vi "ErrorHandler.vi"(6 "EnqueueType (QMH)":T1, 8 "error in (no error)":errorcluster, 11 "Queue Array Reference In":refnum<queue>[](array[refnum])) -> (0 "error out":errorcluster)   [LabVIEW 2018, in "ScopePlugins.lvlib"]
uses:
  ScopePlugins.lvlib
  TypeDefs/QueueNames.ctl
  clMessage.ctl
  EnqueueTypes.ctl
panel:
  in  "Message (Error)":string="Error"
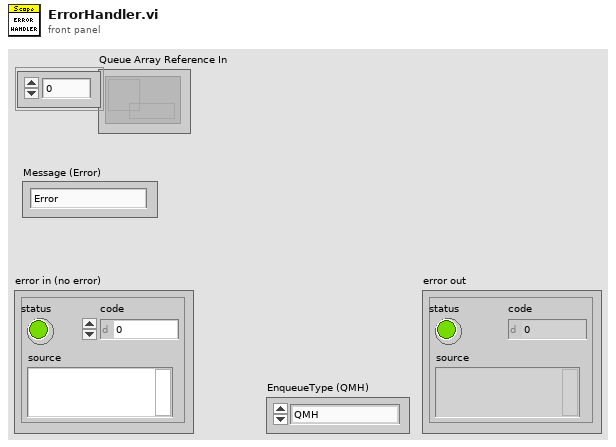
[diagram p1: front panel]
types:
  T1 = typedef "ScopePlugins.lvlib/QueueNames.ctl" = enum16{"QMH", "Class ", "MA"}
  T2 = typedef "ScopePlugins.lvlib/EnqueueTypes.ctl" = enum16{"LossyEnqueue", "EnqueueAtFront", "Enqueue"}
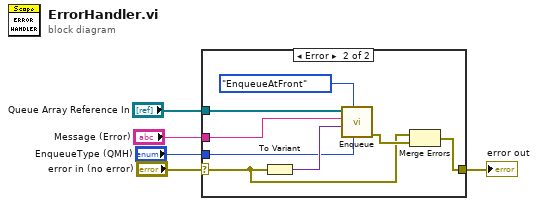
[diagram p0: block diagram]
diagram:
  n1 = case shown="Error" "error in (no error)" {
    selector: "error in (no error)" -> [w6 w7]
    tunnel: "Message (Error)" -> [_ w13]
    tunnel: "Queue Array Reference In" -> [_ w12]
    tunnel: "EnqueueType (QMH)" -> [_ w11]
    tunnel: [w6 w9] -> w2
    frame No Error {
    }
    frame Error {
      n2 = To Variant(anything=w7) -> (Variant=w14:variant)
      n3 = call "Enqueue.vi"("EnqueueType (QMH)"=w11, "EnqueueType (Enqueue)"=EnqueueTypes."EnqueueAtFront", "Message Data"=w14, "Message"=w13, "Queue Array Reference In"=w12) -> ("error out"=w8:errorcluster)  [unwired: 4 in, 2 out]
      n4 = Merge Errors(w7, w8) -> (w9:errorcluster)
    }
  }
  "error out" <- w2
